vi "set_value.vi"() -> ()   [LabVIEW 2019]
uses:
  Global.vi
panel:
  out "spill_id_global":i64
  in  "stop":bool
  out "spill_id":i64
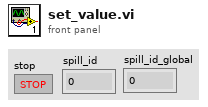
[diagram p1: front panel]
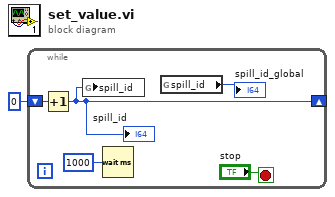
[diagram p0: block diagram]
diagram:
  n1 = while {
    shift-right: [w3] -> _
    shift-left: 0 -> [w6]
    stop <- "stop" stop-if-true
    n2 = Increment(x=w6) -> (x+1=w3:i32)
    "spill_id" <- w3
    n3 = global write "Global.vi" "spill_id"(w3) -> ()
    n4 = Wait (ms)(milliseconds to wait=u32 1000) -> ()  [unwired: 1 out]
    n5 = global read "Global.vi" "spill_id"() -> (→"spill_id_global":i64)
  }
